vi "Scaled Time Domain Window.vi"   [LabVIEW 2012, in "NI_AALPro.lvlib"]
doc: "Applies a scaled window to the input sequence <B>X</B>. Wire data to the <B>X</B> input to determine the polymorphic instance to use or manually select the instance."
uses:
  NI_AALPro.lvlib
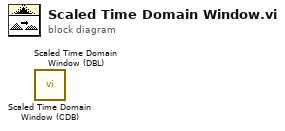
[diagram p0: block diagram]
diagram:
  n1 = call "Scaled Time Domain Window (CDB).vi"() -> ()  [unwired: 9 in, 3 out]
  n2 = call "Scaled Time Domain Window (DBL).vi"() -> ()  [unwired: 9 in, 3 out]
